vi "High Gear Calibrations.vi"() -> ()   [LabVIEW 2016]
panel:
  in  "High Gear Calibrations File Location":path=path "C:/ni-rt/startup/HighGearCalibrations.txt"
  out "Right Drive Integral Gain High Gear":dbl
  out "Right Drive Derivative High Gear":dbl
  out "Right Drive Feed-Forward Gain High Gear":dbl
  out "Left Drive Derivative Gain High Gear":dbl
  out "Left Drive Feed-Forward Gain Low Gear":dbl
  out "Right Drive Proportional Gain High Gear":dbl
  out "Max RPM High Gear":dbl
  out "Left Drive Proportional Gain High Gear":dbl
  out "Left Drive Integral Gain High Gear":dbl
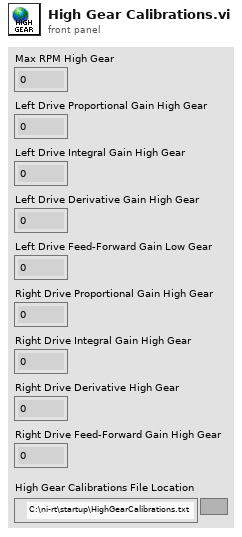
[diagram p1: front panel]
diagram:
